vi "Generate Error.vi"(8 "Error In":errorcluster, 10 "Arguments":string[](array[string]), 11 "Error":T1) -> (0 "Error Out":errorcluster)   [LabVIEW 2013, in "LVH-XBMC.lvlib"]
uses:
  <vilib>/LabVIEW Hacker/XBMC/LVH-XBMC.lvlib
  <vilib>/LabVIEW Hacker/XBMC/Private/Type Defs/Error.ctl
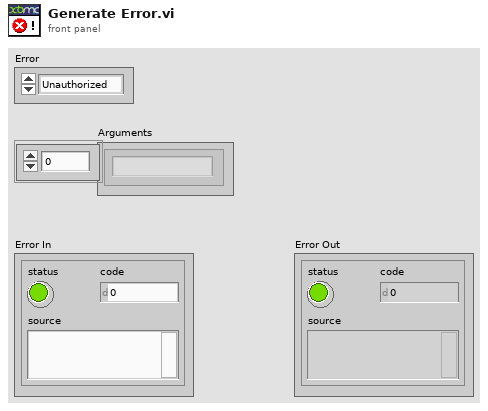
[diagram p1: front panel]
types:
  T1 = typedef "LVH-XBMC.lvlib/Error.ctl" = enum16{"Unauthorized"}
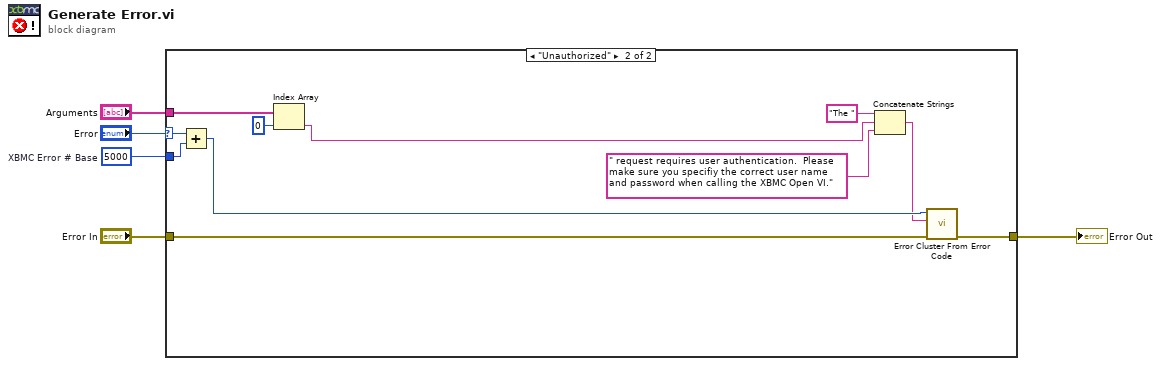
[diagram p0: block diagram]
diagram:
  w1 = 5000  # XBMC Error # Base
  n1 = case shown="\"Unauthorized\"" "Error" {
    selector: "Error" -> [_ w14]
    tunnel: "Error In" -> [w6 w17]
    tunnel: [w6 w16] -> w4
    tunnel: "Arguments" -> [_ w15]
    tunnel: w1 -> [_ w13]
    frame Default {
      # "No Error"
    }
    frame "Unauthorized" {
      n2 = Add(x=w14, y=w13) -> (x+y=w12:i32)
      n3 = Index Array(array=w15, index=0) -> (element=w10:string)
      n4 = Concatenate Strings("The " ("string"), w10, " request requires user authentication.  Please make sure you specifiy the correct user name and password when calling the XBMC Open VI." ("string")) -> (w7:string)
      n5 = call <vilib>:"Error Cluster From Error Code.vi"("error in (no error)"=w17, "error message (\"\")"=w7, "error code (0)"=w12) -> ("error out"=w16:errorcluster)  [unwired: 6 in]
    }
  }
  "Error Out" <- w4
